vi "Update Add Run Subpanel.vi"(8 "error in (no error)":errorcluster, 11 "Scan SBlock in":refnum<class "Scan SBlock.lvclass">) -> (0 "error out":errorcluster, 2 "Subpanel ref":refnum<vi>, 3 "Scan SBlock out":refnum<class "Scan SBlock.lvclass">)   [LabVIEW 2020, in "TALOS.lvlib" / "Run Utilities.lvlib" / "Scan SBlock.lvclass"]
uses:
  Scan SBlock.lvclass
  Scan SBlock.lvclass/Scan SBlock.ctl
  Scan Mode Panel.vi
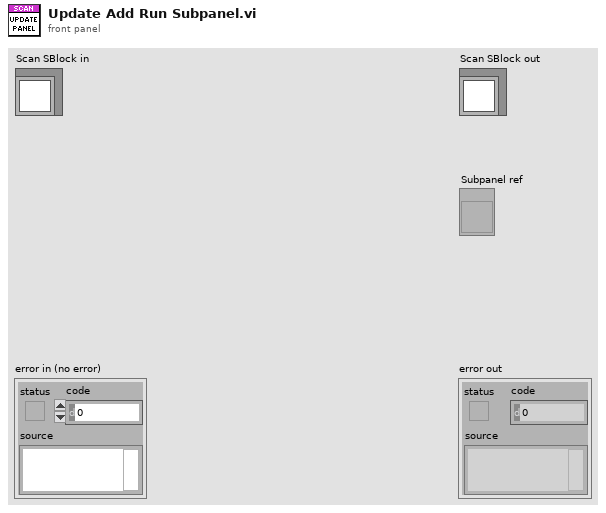
[diagram p1: front panel]
types:
  T1 = typedef "TALOS.lvlib/Run Utilities.lvlib/Scan SBlock.lvclass/Advanced Parameters.ctl" = cluster{"Param":string, "From":dbl, "To":dbl, "Step":dbl, "Mode":T2}
  T2 = typedef "TALOS.lvlib/Run Utilities.lvlib/Scan SBlock.lvclass/Advanced Panel Parameter Mode.ctl" = enum16{"Linear", "Log", "LINKED"}
  T3 = typedef "TALOS.lvlib/Run Utilities.lvlib/Scan SBlock.lvclass/Advanced Parameters - list.ctl" = cluster{"Param":string, "List of values":string[]}
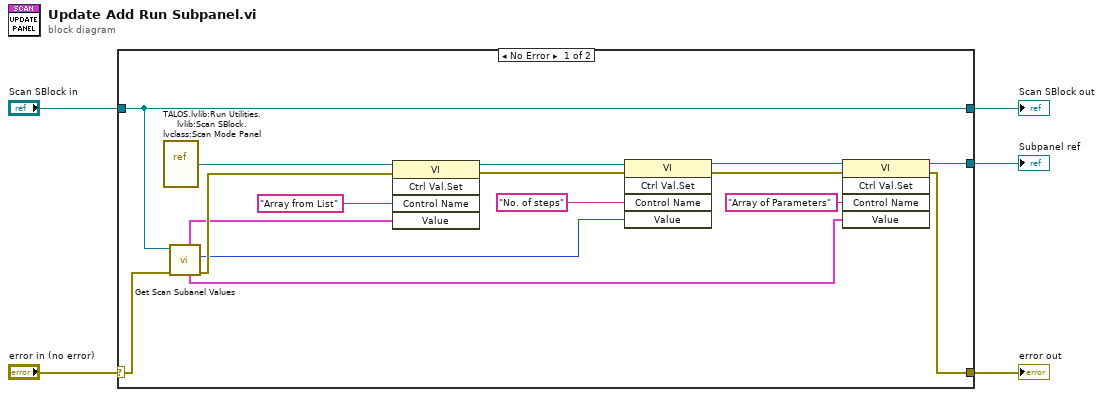
[diagram p0: block diagram]
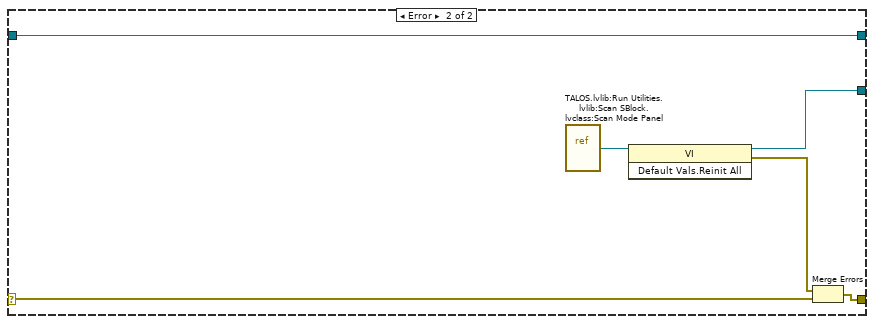
[diagram p2: hidden frame]
diagram:
  n1 = case shown="No Error" "error in (no error)" {
    selector: "error in (no error)" -> [w9 w25]
    tunnel: [w8 w24] -> w4
    tunnel: [w7 w27] -> w2
    tunnel: "Scan SBlock in" -> [w7 w27]
    tunnel: [w6 w22] -> w1
    frame No Error {
      n2 = vi-ref "TALOS.lvlib:Run Utilities.lvlib:Scan SBlock.lvclass:Scan Mode Panel.vi"() -> (w21:refnum<vi>)
      n3 = call-dynamic "Get Scan Subanel Values.vi"("error in (no error)"=w9, "Scan SBlock in"=w7) -> ("error out"=w13:errorcluster, "No. of steps"=w11:u32, "Array of Parameters"=w10:T1[], "Array from List"=w12:T3[])  [unwired: 5 in, 1 out]
      n4 = invoke class="VI" method="Ctrl Val.Set"(reference=w21, error in=w13, "Control Name"="Array from List", "Value"=w12) -> (reference out=w18:refnum<vi>, error out=w16:errorcluster)  [unwired: 1 in, 3 out]
      n5 = invoke class="VI" method="Ctrl Val.Set"(reference=w18, error in=w16, "Control Name"="No. of steps", "Value"=w11) -> (reference out=w15:refnum<vi>, error out=w14:errorcluster)  [unwired: 1 in, 3 out]
      n6 = invoke class="VI" method="Ctrl Val.Set"(reference=w15, error in=w14, "Control Name"="Array of Parameters", "Value"=w10) -> (reference out=w6:refnum<vi>, error out=w8:errorcluster)  [unwired: 1 in, 3 out]
    }
    frame Error {
      n7 = vi-ref "TALOS.lvlib:Run Utilities.lvlib:Scan SBlock.lvclass:Scan Mode Panel.vi"() -> (w26:refnum<vi>)
      n8 = invoke class="VI" method="Default Vals.Reinit All"(reference=w26) -> (reference out=w22:refnum<vi>, error out=w23:errorcluster)  [unwired: 2 in, 1 out]
      n9 = Merge Errors(w23, w25) -> (w24:errorcluster)
    }
  }
  "error out" <- w4
  "Scan SBlock out" <- w2
  "Subpanel ref" <- w1
